vi "ArmSource and TrigMode to Mode (No Obj).vi"(1 "Pulse Mode":enum16{"Pulses", "Pattern"}(ring), 2 "Arming (Trigger) Source (0:Internal PLL)":T1(ring)) -> (0 "Modes (changes immediately)":T2(ring))   [LabVIEW 2009]
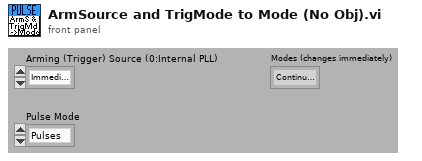
[diagram p1: front panel]
types:
  T1 = enum16{"Immediate (Continuous Mode)", "Internal PLL", "External", "Manual"}
  T2 = enum32{"Continuous Pulsed", "Continuous Pattern", "Internal Triggered Pattern", "External Triggered Pulsed", "External Triggered Pattern", "Other"}
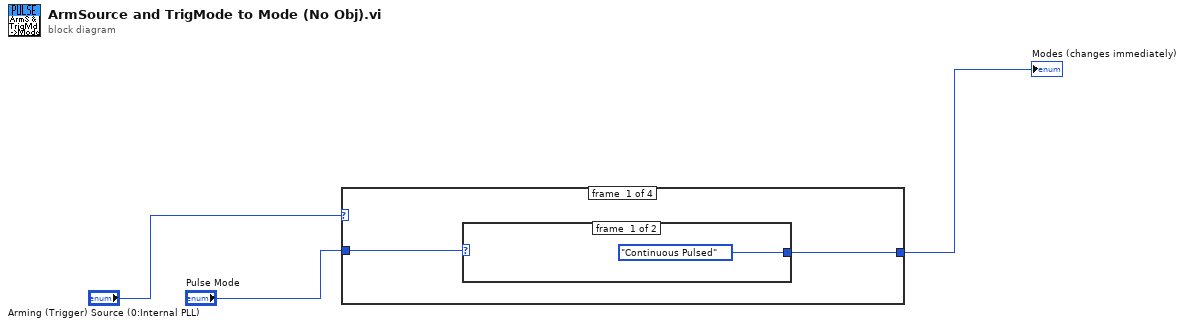
[diagram p0: block diagram]
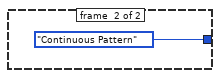
[diagram p2: hidden frame]
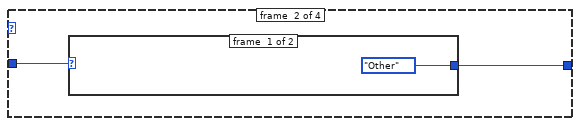
[diagram p3: hidden frame]
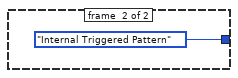
[diagram p4: hidden frame]
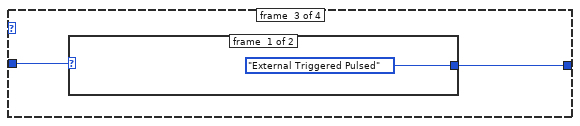
[diagram p5: hidden frame]
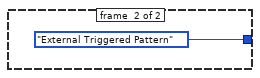
[diagram p6: hidden frame]
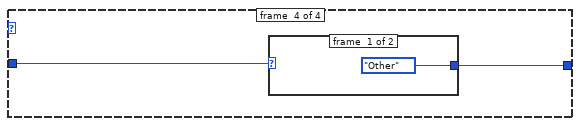
[diagram p7: hidden frame]
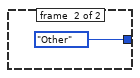
[diagram p8: hidden frame]
diagram:
  n1 = case shown="\"Immediate (Continuous Mode)\", Default" "Arming (Trigger) Source (0:Internal PLL)" {
    tunnel: [w5 w9 w13 w17] -> w2
    tunnel: "Pulse Mode" -> [w4 w8 w12 w16]
    frame #0 {
      n2 = case shown="\"Pulses\", Default" w4 {
        tunnel: [T2."Continuous Pulsed" ("Modes (changes immediately)") T2."Continuous Pattern" ("Modes (changes immediately)")] -> w5
        frame #0 {
        }
        frame #1 {
        }
      }
    }
    frame #1 {
      n3 = case shown="\"Pulses\", Default" w8 {
        tunnel: [T2."Other" ("Modes (changes immediately)") T2."Internal Triggered Pattern" ("Modes (changes immediately)")] -> w9
        frame #0 {
        }
        frame #1 {
        }
      }
    }
    frame #2 {
      n4 = case shown="\"Pulses\", Default" w12 {
        tunnel: [T2."External Triggered Pulsed" ("Modes (changes immediately)") T2."External Triggered Pattern" ("Modes (changes immediately)")] -> w13
        frame #0 {
        }
        frame #1 {
        }
      }
    }
    frame #3 {
      n5 = case shown="\"Pulses\", Default" w16 {
        tunnel: [T2."Other" ("Modes (changes immediately)") T2."Other" ("Modes (changes immediately)")] -> w17
        frame #0 {
        }
        frame #1 {
        }
      }
    }
  }
  "Modes (changes immediately)" <- w2
